vi "setPenWidthF.vi"(8 "Error In":errorcluster, 10 "width":dbl, 11 "QwtAbstractScaleDraw In":refnum<class "QwtAbstractScaleDraw.lvclass">) -> (0 "Error Out":errorcluster, 3 "QwtAbstractScaleDraw Out":refnum<class "QwtAbstractScaleDraw.lvclass">)   [LabVIEW 2014, in "QwtAbstractScaleDraw.lvclass"]
doc: "LabVIEW-specific documentation is not yet available. See <b>https://qwt.sourceforge.io/class_qwt_abstract_scale_draw.html#setPenWidthF</b>"
uses:
  QwtAbstractScaleDraw.lvclass
  LQ Core/LQIdentity/LQIdentity.lvclass/LQIdentity.ctl
  LQ Core/LQ Core.lvlib
  LQ Core/LQIdentity/LQIdentity.lvclass
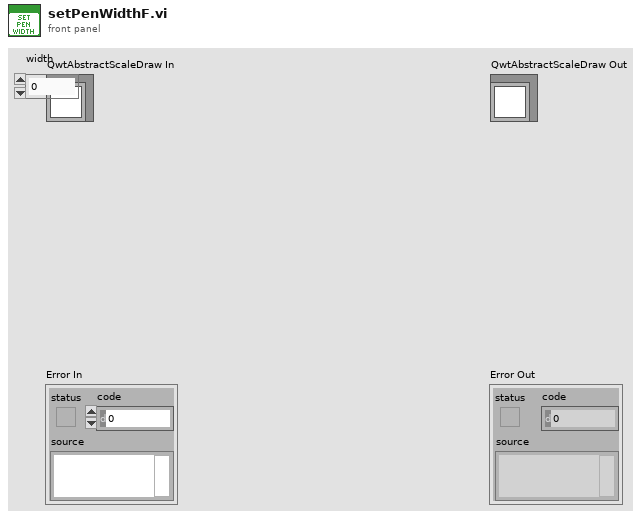
[diagram p1: front panel]
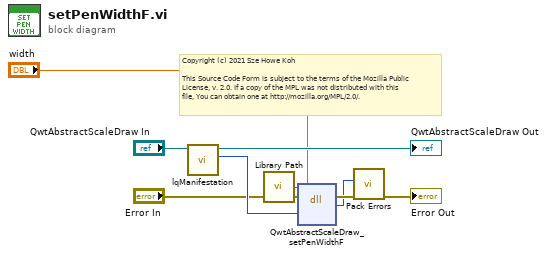
[diagram p0: block diagram]
diagram:
  # "Copyright (c) 2021 Sze Howe Koh\n\nThis Source Code Form is subject to the terms of the Mozilla Public\nLicense, v. 2.0. If a copy of the MPL was not distributed with this\nfile, You can obtain one at http://mozilla.org/MPL/2.0/."
  n1 = call "lqManifestation.vi"("LQIdentity in"="QwtAbstractScaleDraw In") -> ("Manifestation"=w6:u64, "LQIdentity out"=→"QwtAbstractScaleDraw Out":refnum<class "QwtAbstractScaleDraw.lvclass">)  [unwired: 9 in]
  n2 = call "Library Path.vi"() -> ("Library Path"=w7:path)
  n3 = dll-call lib="?" fn="QwtAbstractScaleDraw_setPenWidthF"(path in=w7, error in="Error In", "_instance"=w6, "width"="width") -> (error out=w4:errorcluster, w2:i32)  [unwired: 3 in, 1 out]
  n4 = call "Pack Errors.vi"("Error In"=w4, "Error Code"=w2) -> ("Error Out"=→"Error Out":errorcluster)  [unwired: 9 in]
